vi "Acq_audio_signal.vi"() -> ()   [LabVIEW 2024]
uses:
  <vilib>/Analysis/4window.llb/windowTd.ctl
  <vilib>/sound2/lvsound2.llb/Sound Data Format.ctl
  <vilib>/sound2/lvsound2.llb/Sampling Mode.ctl
  <vilib>/sound2/lvsound2.llb/Sound File Write Open.vi
  <vilib>/sound2/lvsound2.llb/Sound Input Read (DBL).vi
  <vilib>/sound2/lvsound2.llb/Sound File Write (DBL).vi
  <vilib>/measure/maspectr.llb/FFT Power Spectrum and PSD for N Chan.vi
  <vilib>/measure/NI_MAPro.lvlib
  <vilib>/Analysis/NI_AALPro.lvlib
panel:
  in  "path":path
  in  "window":T1=1 items=["Rectangle"=0, "Hanning"=1, "Hamming"=2, "Blackman-Harris"=3, "Exact Blackman"=4, "Blackman"=5, "Flat Top"=6, "4 Term B-Harris "=7, "7 Term B-Harris"=8, "Low Sidelobe"=9, "Blackman Nuttall"=11, "Triangle"=30, "Bartlett-Hanning"=31, "Bohman"=32, "Parzen"=33, "Welch"=34, "Kaiser"=60, "Dolph-Chebyshev"=61, "Gaussian"=62]
  in  "dB":bool
  out "Waveform Graph":cluster{"f0":dbl, "df":dbl, "magnitude":dbl[]}[](graph)
  out "Waveform Graph 2":waveform(dbl)[](graph)
  in  "?":bool
  in  "number of samples/ch":i32=10000
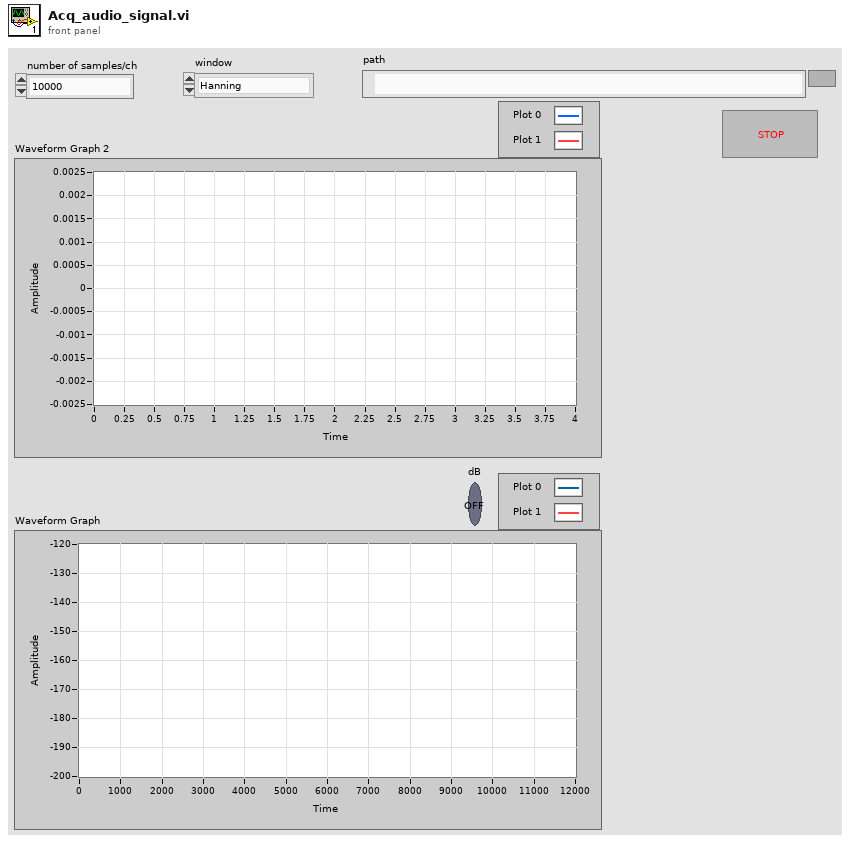
[diagram p1: front panel]
types:
  T1 = typedef "NI_AALPro.lvlib/windowTd.ctl" = u32
  T2 = typedef "Sampling Mode.ctl" = i32
  T3 = typedef "Sound Data Format.ctl" = cluster{"sample rate (S/s)":dbl, "number of channels":i32, "bits per sample":i32}
  T4 = typedef "Sound Input Task ID.ctl" = u32
  T5 = typedef "Sound File Refnum.ctl" = refnum<file>
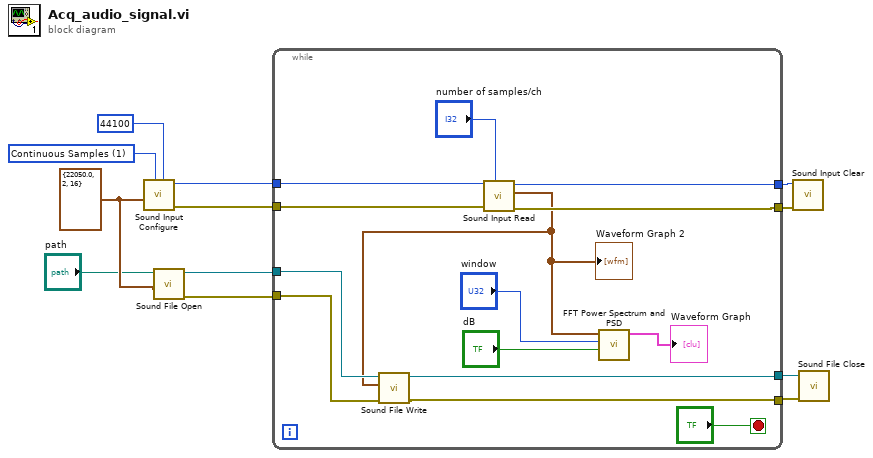
[diagram p0: block diagram]
diagram:
  w12 = T2 1 items=["Finite Samples", "Continuous Samples"] ("sample mode")
  w4 = T3 {"sample rate (S/s)"=22050.0, "number of channels"=2, "bits per sample"=16} ("sound format")
  n1 = call <vilib>:"Sound Input Configure.vi"("number of samples/ch"=44100, "sample mode"=w12, "sound format"=w4) -> ("error out"=w10:errorcluster, "task ID"=w9:T4)  [unwired: 7 in]
  n2 = call-poly <vilib>:"Sound File Open.vi"("sound format"=w4, "path"="path") -> ("error out"=w5:errorcluster, "sound file refnum"=w6:T5)  [unwired: 8 in]
  n3 = while {
    tunnel: w10 -> [w26]
    tunnel: [w23] -> w7
    tunnel: [w22] -> w8
    tunnel: w9 -> [w21]
    tunnel: w6 -> [w17]
    tunnel: w5 -> [w16]
    tunnel: [w14] -> w3
    tunnel: [w13] -> w2
    stop <- "?" stop-if-true
    n4 = call-poly <vilib>:"Sound Input Read.vi"("number of samples/ch"="number of samples/ch", "error in (no error)"=w26, "task ID"=w21) -> ("error out"=w23:errorcluster, "data"=w15:waveform(dbl)[], "task ID out"=w22:T4)  [unwired: 6 in]
    "Waveform Graph 2" <- w15
    n5 = call-poly <vilib>:"Sound File Write.vi"("error in (no error)"=w16, "data"=w15, "sound file refnum"=w17) -> ("error out"=w13:errorcluster, "sound file refnum out"=w14:T5)  [unwired: 7 in]
    n6 = call-poly <vilib>:"FFT Power Spectrum and PSD.vi"("dB On (F)"="dB", "window"="window", "time signals"=w15) -> ("Power Spectrum / PSD"=→"Waveform Graph":cluster{"f0":dbl, "df":dbl, "magnitude":dbl[]}[])  [unwired: 5 in, 3 out]
  }
  n7 = call <vilib>:"Sound Input Clear.vi"("error in (no error)"=w7, "task ID"=w8) -> ()  [unwired: 9 in, 1 out]
  n8 = call <vilib>:"Sound File Close.vi"("error in (no error)"=w2, "sound file refnum"=w3) -> ()  [unwired: 9 in, 1 out]
